vi "Start.vi"(9 "Alias":string, 10 "Actor":refnum<class "Actor.lvclass">, 11 "Base Actor in":refnum<class "Base Actor.lvclass">) -> (0 "Error out":errorcluster, 3 "Base Actor out":refnum<class "Base Actor.lvclass">)   [LabVIEW 2025, in "jettl.lvlib" / "Actor.lvlib" / "Base Actor.lvclass"]
uses:
  Base Actor.lvclass
  Actor/Actor.lvclass
  Attributes/Attributes/Attributes.lvclass
  Queues.ctl
  Config Actor.ctl
  Base Actor.lvclass/Base Actor.ctl
  Actor.lvlib
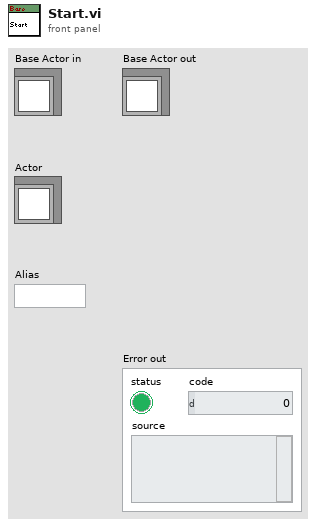
[diagram p1: front panel]
types:
  T1 = typedef "jettl.lvlib/Actor.lvlib/Config Actor.ctl" = cluster{"Alias":string, "Creator Attributes":refnum<class "Attributes.lvclass">, "Queues":T2}
  T2 = typedef "jettl.lvlib/Actor.lvlib/Queues.ctl" = cluster{"Self Attributes":refnum<queue>, "Error":refnum<queue>}
  T3 = typedef "jettl.lvlib/Actor.lvlib/Base Actor.lvclass/Created Attributes Map.ctl" = map{string, refnum<class "Attributes.lvclass">}
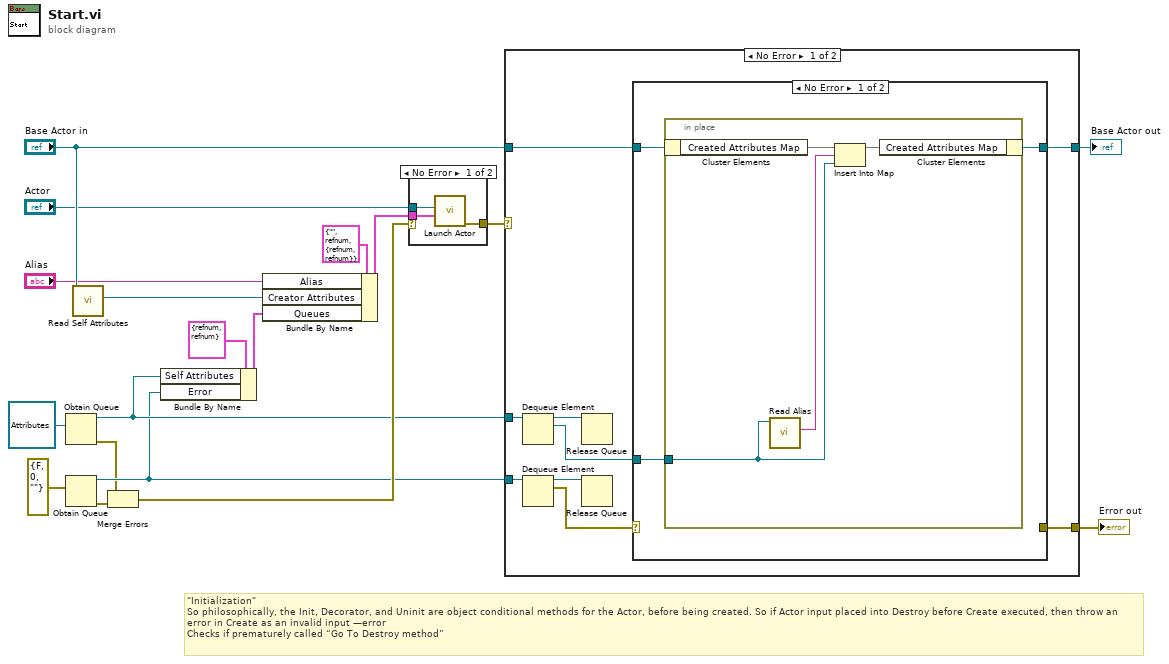
[diagram p0: block diagram]
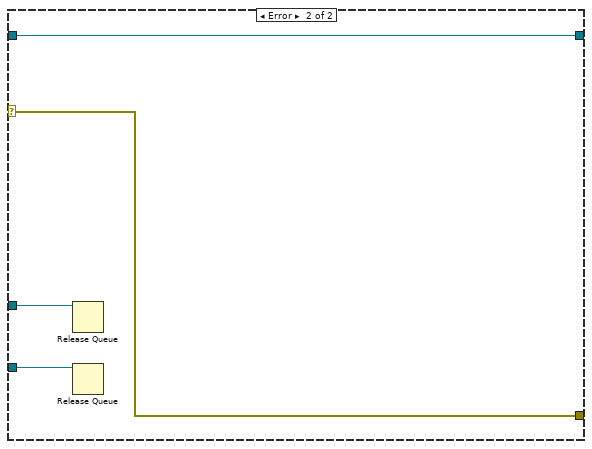
[diagram p3: hidden frame]
diagram:
  # "\"Initialization\"\nSo philosophically, the Init, Decorator, and Uninit are object conditional methods for the Actor, before being created. So if Actor input placed into Destroy before Create executed, then throw an error in Create as an invalid input —error  \nChecks if prematurely called “Go To Destroy method”"
  n1 = Obtain Queue(element data type=refnum<class "Attributes.lvclass"> refnum ("jettl.lvlib:Attributes.lvlib:Attributes.lvclass")) -> (queue out=w10:refnum<queue>, error out=w8:errorcluster)  [unwired: 4 in, 1 out]
  n2 = Obtain Queue(element data type=errorcluster {"status"=FALSE, "code"=0, "source"=""} ("Error")) -> (queue out=w9:refnum<queue>, error out=w7:errorcluster)  [unwired: 4 in, 1 out]
  n3 = call-dynamic "Read Self Attributes.vi"("Base Actor in"="Base Actor in") -> ("Self Attributes"=w4:refnum<class "Attributes.lvclass">)  [unwired: 10 in]
  n4 = Merge Errors(w8, w7) -> (w12:errorcluster)
  n5 = Bundle By Name(cluster=T2 {"Self Attributes"=refnum, "Error"=refnum} ("Queues"), "Self Attributes"=w10, "Error"=w9) -> (w3:T2)
  n6 = Bundle By Name(cluster=T1 {"Alias"="", "Creator Attributes"=refnum, "Queues"={"Self Attributes"=refnum, "Error"=refnum}} ("Config Actor"), "Alias"="Alias", "Creator Attributes"=w4, "Queues"=w3) -> (w1:T1)
  n7 = case shown="No Error" w12 {
    selector: w12 -> [_ w22]
    tunnel: [w21 w22] -> w15
    tunnel: "Actor" -> [w20 _]
    tunnel: w1 -> [w19 _]
    frame No Error {
      n8 = call "Launch Actor.vi"("Config Actor"=w19, "Actor"=w20) -> ("Error out"=w21:errorcluster)  [unwired: 9 in]
    }
    frame Error {
    }
  }
  n9 = case shown="No Error" w15 {
    selector: w15 -> [_ w41]
    tunnel: "Base Actor in" -> [w31 w43]
    tunnel: [w30 w43] -> w18
    tunnel: w10 -> [w29 w44]
    tunnel: w9 -> [w27 w42]
    tunnel: [w23 w41] -> w16
    frame No Error {
      n10 = Dequeue Element(queue=w29) -> (queue out=w28:refnum<queue>, element=w25:refnum<class "Attributes.lvclass">)  [unwired: 2 in, 2 out]
      n11 = Dequeue Element(queue=w27) -> (queue out=w26:refnum<queue>, element=w24:errorcluster)  [unwired: 2 in, 2 out]
      n12 = Release Queue(queue=w28) -> ()  [unwired: 2 in, 3 out]
      n13 = Release Queue(queue=w26) -> ()  [unwired: 2 in, 3 out]
      n14 = case shown="No Error" w24 {
        selector: w24 -> [_ w39]
        tunnel: w31 -> [w33 w40]
        tunnel: [w32 w40] -> w30
        tunnel: w25 -> [w34 _]
        tunnel: [_ w39] -> w23
        frame No Error {
          n15 = in-place {
            in-place-border: w34 -> [w35]
            n16 = in-place-cluster #1(w33) -> ("Created Attributes Map"=w38:T3)
            n17 = call-dynamic "Read Alias.vi"("Attributes in"=w35) -> ("Alias"=w36:string)  [unwired: 10 in]
            n18 = Insert Into Map(map in=w38, key=w36, value=w35) -> (map out=w37:T3)  [unwired: 2 out]
            n19 = in-place-cluster #1("Created Attributes Map"=w37) -> (w32:refnum<class "Base Actor.lvclass">)
          }
        }
        frame Error {
        }
      }
    }
    frame Error {
      n20 = Release Queue(queue=w44) -> ()  [unwired: 2 in, 3 out]
      n21 = Release Queue(queue=w42) -> ()  [unwired: 2 in, 3 out]
    }
  }
  "Base Actor out" <- w18
  "Error out" <- w16
